vi "Marker Bandwidth Search Result.vi"(5 "Marker (1)":i32=1, 7 "Channel (1)":i32=1, 8 "error in (no error)":errorcluster, 11 "VISA resource name":refnum<visa-resource-name>) -> (0 "error out":errorcluster, 1 "Loss":dbl format="%^.2e", 2 "Bandwidth":dbl format="%^.2e", 3 "VISA resource name out":refnum<visa-resource-name>, 4 "Q Value":dbl format="%^.2e", 6 "Center Frequency":dbl format="%^.2e")   [LabVIEW 2022 SP3, in "Agilent ENA Series.lvlib"]
doc: "Reads out the bandwidth search result of selected marker, for the active trace of selected channel."
uses:
  <instrlib>/VNA/Agilent ENA Series/Agilent ENA Series.lvlib
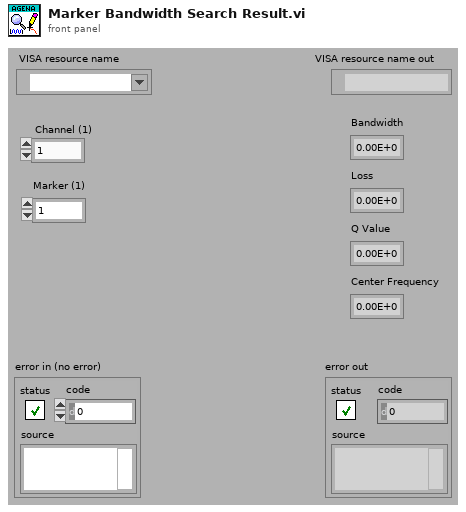
[diagram p1: front panel]
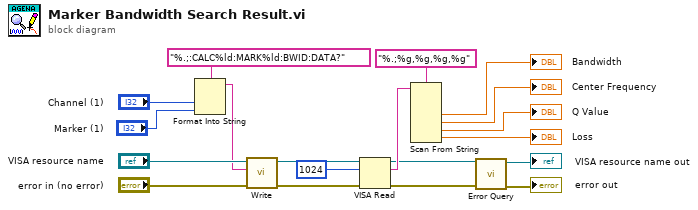
[diagram p0: block diagram]
diagram:
  n1 = Format Into String(format string="%.;:CALC%ld:MARK%ld:BWID:DATA?", "Channel (1)", "Marker (1)") -> (resulting string=w10:string)  [unwired: 2 in, 1 out]
  n2 = call <instrlib>:"Write.vi"("error in (no error)"="error in (no error)", "String ()"=w10, "VISA resource name"="VISA resource name") -> ("error out"=w16:errorcluster, "VISA resource name out"=w17:refnum<visa-resource-name>)  [unwired: 6 in, 1 out]
  n3 = VISA Read(VISA resource name=w17, byte count=u32 1024, error in (no error)=w16) -> (VISA resource name out=w4:refnum<visa-resource-name>, read buffer=w14:string, error out=w3:errorcluster)  [unwired: 1 out]
  n4 = Scan From String(format string="%.;%g,%g,%g,%g", input string=w14) -> (output 1=→"Bandwidth":dbl, output 2=→"Center Frequency":dbl, output 3=→"Q Value":dbl, output 4=→"Loss":dbl)  [unwired: 6 in, 3 out]
  n5 = call <instrlib>:"Error Query.vi"("error in (no error)"=w3, "VISA resource name"=w4) -> ("error out"=→"error out":errorcluster, "VISA resource name out"=→"VISA resource name out":refnum<visa-resource-name>)  [unwired: 6 in, 2 out]
